vi "EstimatePlaneForPointSet.vi"(8 "error in":errorcluster, 11 "Point Set":T1[](array[typedef])) -> (0 "error out":errorcluster, 1 "Points  Centred Around Mean Point":dbl[][](array[numeric]), 2 "Mean Point":dbl[](array[numeric]), 3 "Plane Coeffcients":T2)   [LabVIEW 2020, in "pointset_utils.lvlib" / "Align Point Set to Plane.lvlib"]
uses:
  Align Point Set to Plane.lvlib
  PlaneCoeffecients.ctl
  common/Object Point (Float).ctl
  <vilib>/Analysis/7linalg.llb/SVD Option.ctl
  <vilib>/Analysis/baseanly.llb/Mean (DBL).vi
  <vilib>/Analysis/baseanly.llb/Real Dot Product.vi
  <vilib>/Analysis/7linalg.llb/Real SVD Decomposition.vi
  <vilib>/Analysis/NI_AALPro.lvlib
  <vilib>/Analysis/NI_AALBase.lvlib
  common/common.lvlib
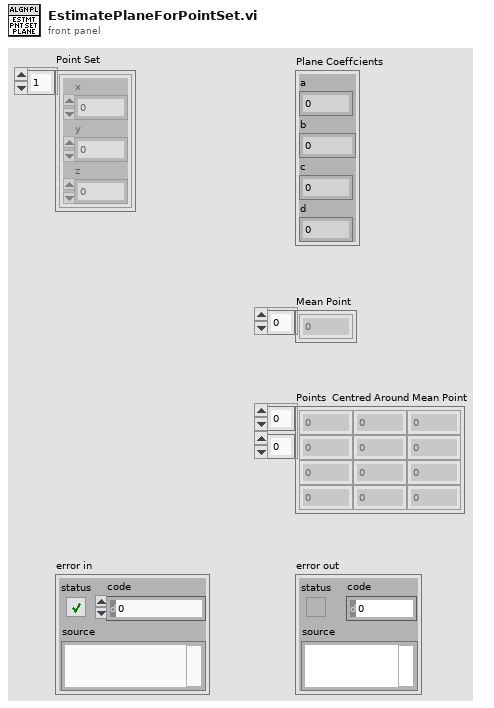
[diagram p1: front panel]
types:
  T1 = typedef "common.lvlib/Object Point (Float).ctl" = cluster{"x":dbl, "y":dbl, "z":dbl}
  T2 = typedef "pointset_utils.lvlib/Align Point Set to Plane.lvlib/PlaneCoeffecients.ctl" = cluster{"a":dbl, "b":dbl, "c":dbl, "d":dbl}
  T3 = typedef "NI_AALPro.lvlib/SVD Option.ctl" = u16
  T4 = typedef "NI_Matrix.lvlib/RealMatrix.ctl" = dbl[][]
  T5 = cluster{"[0]":dbl, "[1]":dbl, "[2]":dbl, "[3]":dbl}
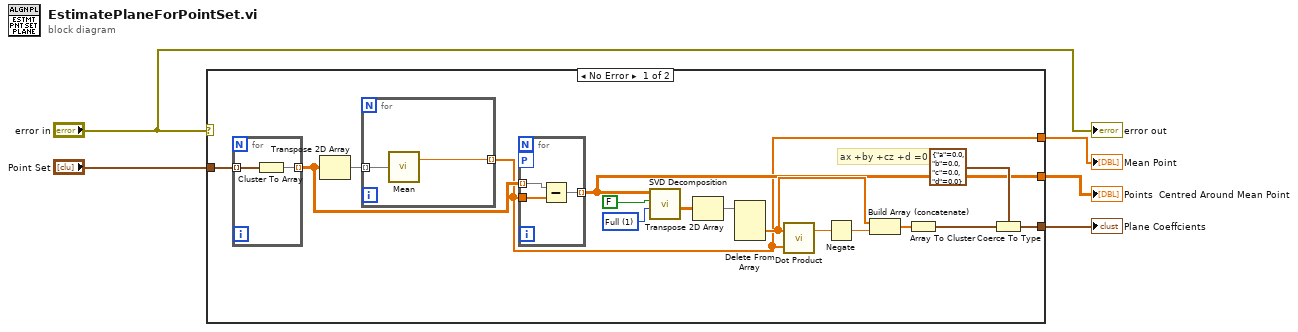
[diagram p0: block diagram]
diagram:
  n1 = case shown="No Error" "error in" {
    tunnel: [w11 _] -> w5
    tunnel: [w10 _] -> w4
    tunnel: "Point Set" -> [w9 _]
    tunnel: [w6 _] -> w2
    frame No Error {
      w14 = T3 1 items=["Thin", "Full"] ("SVD option")
      # "ax +by +cz +d =0"
      n2 = for {
        tunnel: w9 -> [w23] mode=indexing
        tunnel: [w22] -> w7 mode=indexing
        n3 = Cluster To Array(cluster=w23) -> (array=w22:dbl[])
      }
      n4 = Transpose 2D Array(2D array=w7) -> (transposed array=w8:dbl[][])
      n5 = for {
        tunnel: w8 -> [w27] mode=indexing
        tunnel: [w28] -> w6 mode=indexing
        n6 = call-poly <vilib>:"Mean.vi"("X"=w27) -> ("mean"=w28:dbl)  [unwired: 1 out]
      }
      n7 = for {
        workers-P: _ -> [_]
        tunnel: w7 -> [w26] mode=indexing
        tunnel: w6 -> [w25]
        tunnel: [w24] -> w11 mode=indexing
        n8 = Subtract(x=w26, y=w25) -> (x-y=w24:dbl[])
      }
      n9 = call-poly <vilib>:"SVD Decomposition.vi"("SVD option"=w14, "singular values only?"=FALSE, "A"=w11) -> ("Matrix V"=w17:T4)  [unwired: 4 in, 4 out]
      n10 = Transpose 2D Array(2D array=w17) -> (transposed array=w12:T4)
      n11 = Delete From Array(array=w12) -> (deleted portion=w13:dbl[])  [unwired: 3 in, 1 out]
      n12 = call-poly <vilib>:"Dot Product.vi"("Y Vector"=w6, "X Vector"=w13) -> ("X * Y"=w19:dbl)  [unwired: 1 out]
      n13 = Negate(x=w19) -> (-x=w21:dbl)
      n14 = Build Array (concatenate)(w13, w21) -> (w18:dbl[])
      n15 = Array To Cluster(array=w18) -> (cluster=w15:T5)
      n16 = Coerce To Type(0:w15, 1:T2 {"a"=0.0, "b"=0.0, "c"=0.0, "d"=0.0}) -> (2:w10:T2)
    }
    frame Error {
    }
  }
  "Plane Coeffcients" <- w4
  "Points  Centred Around Mean Point" <- w5
  "Mean Point" <- w2
  "error out" <- "error in"
